vi "Servo_Write_Intg.vi"(0 "LINX Resource in":T1, 5 "Servo X":dbl(knob)=0.06694852218519998 scale=-48.75..48.75, 7 "Servo Y":dbl(knob)=-0.4415528564582303 scale=-60.0..60.0, 9 "Reset":bool, 11 "error in (no error)":errorcluster) -> (4 "LINX Resource out":T1, 15 "error out":errorcluster)   [LabVIEW 2021]
uses:
  <vilib>/MakerHub/LINX/Private/Type Defs/LINX Ref.ctl
  <vilib>/MakerHub/LINX/Private/Type Defs/Platform.ctl
  <vilib>/MakerHub/LINX/Private/Type Defs/Interface.ctl
  <vilib>/MakerHub/LINX/Private/Device/Type Defs/LINX Device Config.ctl
  <vilib>/MakerHub/LINX/Private/Device/Type Defs/TCP Config.ctl
  <vilib>/MakerHub/LINX/Private/Device/Type Defs/Channels.ctl
  <vilib>/MakerHub/LINX/Public/Sensors/Motion/Servo/Servo Set Pulse Width One Channel.vi
  <vilib>/MakerHub/LINX/Public/Sensors/Motion/Servo/Servo.lvlib
  <vilib>/MakerHub/LINX/LMH-LINX.lvlib
  <vilib>/MakerHub/LINX/Private/Device/Device.lvlib
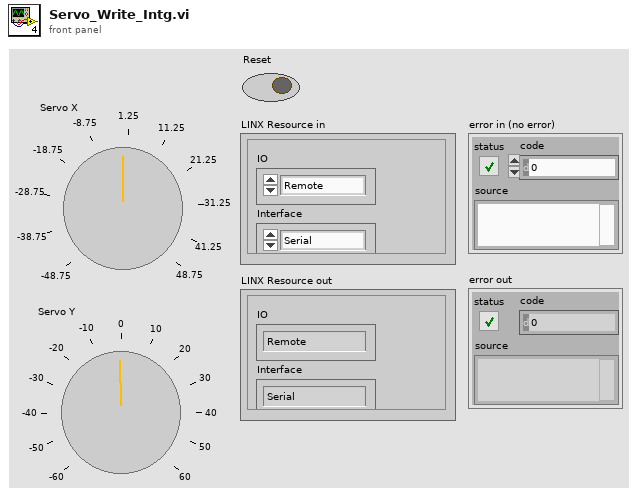
[diagram p1: front panel]
types:
  T1 = typedef "LMH-LINX.lvlib/LINX Ref.ctl" = cluster{"IO":T2, "Interface":T3, "LINX Device Config":T4}
  T2 = typedef "LMH-LINX.lvlib/Platform.ctl" = enum16{"Remote", "Local"}
  T3 = typedef "LMH-LINX.lvlib/Interface.ctl" = enum16{"Serial", "TCP"}
  T4 = typedef "LMH-LINX.lvlib/Device.lvlib/LINX Device Config.ctl" = cluster{"Interface":T3, "COM Port":refnum<visa-resource-name>, "TCP Configuration":T5, "Device Family":u8, "Device ID":u8, "Device Name":string, "TCP Ref":refnum<k5>, "Channels":T6}
  T5 = typedef "LMH-LINX.lvlib/Device.lvlib/TCP Config.ctl" = cluster{"IP Address":string, "Port":u16}
  T6 = typedef "LMH-LINX.lvlib/Channels.ctl" = cluster{"DI":u8[], "DO":u8[], "AI":u8[], "AO":u8[], "PWM":u8[], "QE":u8[], "UART":u8[], "I2C 2":u8[], "SPI":u8[], "CAN":u8[], "Servo":u8[], "AI Ref (V)":dbl, "AI Resolution (Bits)":u8, "AO Ref (V)":dbl, "AO Resolution (Bits)":u8}
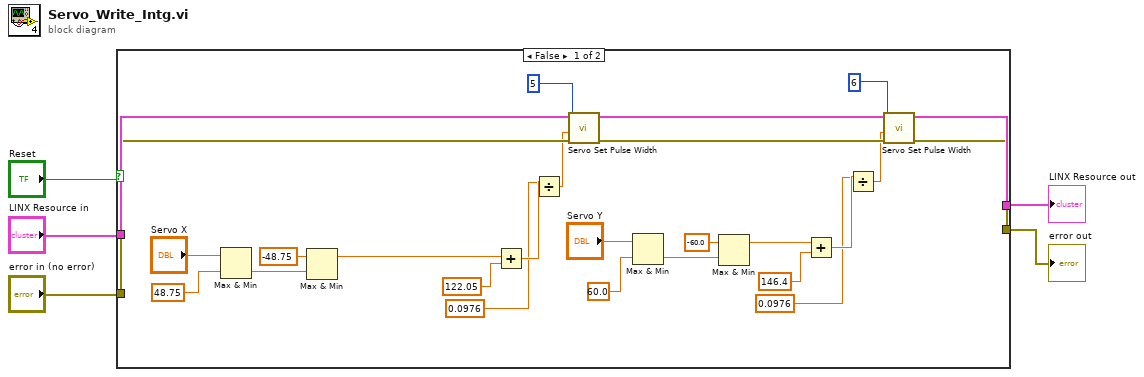
[diagram p0: block diagram]
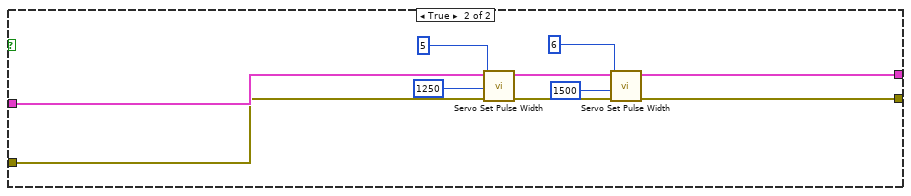
[diagram p2: hidden frame]
diagram:
  n1 = case shown="False" "Reset" {
    tunnel: "LINX Resource in" -> [w29 w41]
    tunnel: [w28 w39] -> w2
    tunnel: "error in (no error)" -> [w27 w38]
    tunnel: [w26 w36] -> w1
    frame False {
      n2 = Max & Min(x="Servo X", y=48.75) -> (min(x,y)=w13:dbl)  [unwired: 1 out]
      n3 = Max & Min(x=-48.75, y=w13) -> (max(x,y)=w11:dbl)  [unwired: 1 out]
      n4 = Add(x=w11, y=122.05) -> (x+y=w22:dbl)
      n5 = Divide(x=w22, y=0.0976) -> (x/y=w20:dbl)
      n6 = call-poly <vilib>:"Servo Set Pulse Width.vi"("Error In"=w27, "Pulse Width (uS)"=w20, "Servo Channel"=u8 5, "LINX Resource"=w29) -> ("Error Out"=w30:errorcluster, "LINX Resource"=w31:T1)  [unwired: 6 in]
      n7 = Max & Min(x="Servo Y", y=60.0) -> (min(x,y)=w10:dbl)  [unwired: 1 out]
      n8 = Max & Min(x=-60.0, y=w10) -> (max(x,y)=w6:dbl)  [unwired: 1 out]
      n9 = Add(x=w6, y=146.4) -> (x+y=w18:dbl)
      n10 = Divide(x=w18, y=0.0976) -> (x/y=w16:dbl)
      n11 = call-poly <vilib>:"Servo Set Pulse Width.vi"("Error In"=w30, "Pulse Width (uS)"=w16, "Servo Channel"=u8 6, "LINX Resource"=w31) -> ("Error Out"=w26:errorcluster, "LINX Resource"=w28:T1)  [unwired: 6 in]
    }
    frame True {
      n12 = call-poly <vilib>:"Servo Set Pulse Width.vi"("Error In"=w38, "Pulse Width (uS)"=u16 1250, "Servo Channel"=u8 5, "LINX Resource"=w41) -> ("Error Out"=w37:errorcluster, "LINX Resource"=w40:T1)  [unwired: 6 in]
      n13 = call-poly <vilib>:"Servo Set Pulse Width.vi"("Error In"=w37, "Pulse Width (uS)"=u16 1500, "Servo Channel"=u8 6, "LINX Resource"=w40) -> ("Error Out"=w36:errorcluster, "LINX Resource"=w39:T1)  [unwired: 6 in]
    }
  }
  "LINX Resource out" <- w2
  "error out" <- w1
